vi "Object Node Tree.vi"(4 "Maximum Depth":i32=-1, 6 "Initial Path":string="$", 8 "error in (no error)":errorcluster, 10 "Offset":i32, 11 "JSON":string) -> (0 "error out":errorcluster, 1 "<JSON>":string[](array[string]) caption="<JSON>Items", 3 "$Paths":string[](array[string]))   [LabVIEW 2020]
doc: "Takes a JSON Value and \"flattens\" the Object structure, producing out arrays of the $Paths to each item and the corresponding items. This works recursively on all subObjects.\n\nNote: to support names containing periods (.) in them, those names will be retuurned as a JSON string (quoted). \n\nFor example: the JSON {\"A\":{\"B1\":1\"B2:\"x\"},\"A2\":true,\"A.1\":{\"C\":123}} produces the arrays:\n$Paths (Items):\n$.A.B1 (1)\n$.A.B2 (\"x\")\n$.A2 (true)\n$.\"A.1\".C (123)"
uses:
  <vilib>/JDP Science/JSONtext/JSONtext.lvlib
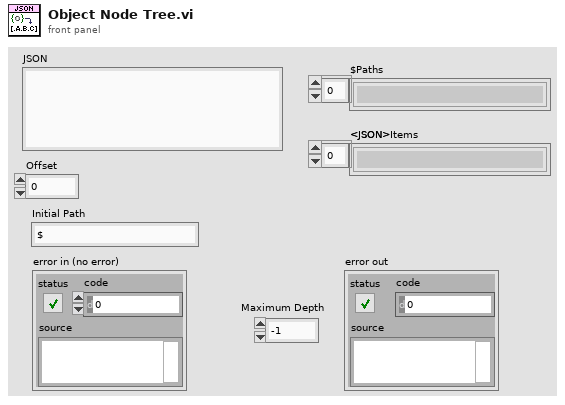
[diagram p1: front panel]
types:
  T1 = typedef "JSONtext.lvlib/JSON Value Type.ctl" = enum16{"Not a JSON Value", "JSON Object", "JSON Array", "String", "Number", "true", "false", "null"}
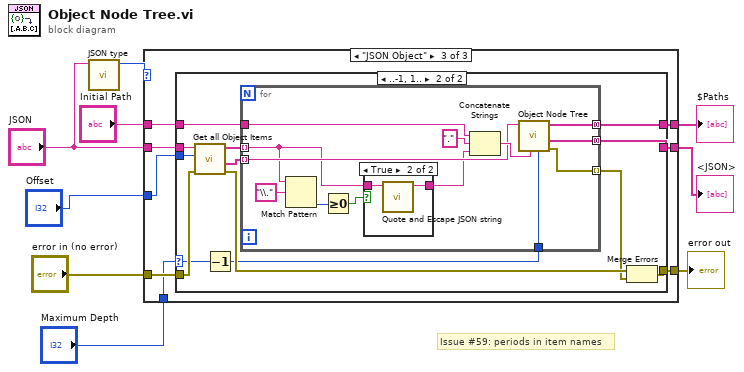
[diagram p0: block diagram]
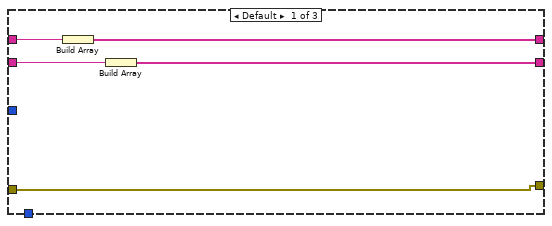
[diagram p2: hidden frame]
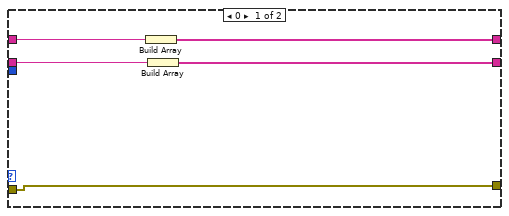
[diagram p4: hidden frame]
diagram:
  # "Issue #59: periods in item names"
  n1 = call <vilib>:"JSON type.vi"("JSON"="JSON") -> ("JSON Value Type"=w5:T1)  [unwired: 9 in, 1 out]
  n2 = case shown="\"JSON Object\"" w5 {
    tunnel: "JSON" -> [w14 _ w23]
    tunnel: [w11 _ w21] -> w6
    tunnel: [w13 _ w20] -> w7
    tunnel: "Initial Path" -> [w12 _ w22]
    tunnel: "Offset" -> [_ _ w19]
    tunnel: "error in (no error)" -> [w10 w15 w18]
    tunnel: [w10 w15 w17] -> w2
    tunnel: "Maximum Depth" -> [_ _ w16]
    frame Default {
      n3 = Build Array(w12) -> (w11:string[])
      n4 = Build Array(w14) -> (w13:string[])
    }
    frame "Not a JSON Value" {
    }
    frame "JSON Object" {
      n5 = case shown="..-1, 1.." w16 {
        selector: w16 -> [_ w30]
        tunnel: w23 -> [w26 w41]
        tunnel: w22 -> [w28 w40]
        tunnel: [w27 w39] -> w21
        tunnel: [w25 w36] -> w20
        tunnel: w19 -> [_ w35]
        tunnel: w18 -> [w24 w34]
        tunnel: [w24 w32] -> w17
        frame 0 {
          n6 = Build Array(w28) -> (w27:string[])
          n7 = Build Array(w26) -> (w25:string[])
        }
        frame ..-1, 1.. {
          n8 = call <vilib>:"Get all Object Items.vi"("error in (no error)"=w34, "Offset"=w35, "JSON"=w41) -> ("error out"=w33:errorcluster, "<JSON>"=w37:string[], "Item Names"=w38:string[])  [unwired: 5 in, 1 out]
          n9 = Decrement(x=w30) -> (x-1=w29:i32)
          n10 = for {
            tunnel: w40 -> [w54]
            tunnel: [w52] -> w39 mode=concatenating
            tunnel: w38 -> [w45] mode=indexing
            tunnel: w37 -> [w50] mode=indexing
            tunnel: [w49] -> w36 mode=concatenating
            tunnel: [w48] -> w31 mode=indexing
            tunnel: w29 -> [w42]
            n11 = Match Pattern(string=w45, regular expression="\\.") -> (offset past match=w46:i32)  [unwired: 1 in, 3 out]
            n12 = Greater Or Equal To 0?(x=w46) -> (x >= 0?=w43:bool)
            n13 = case shown="True" w43 {
              tunnel: w45 -> [w55 w57]
              tunnel: [w55 w56] -> w44
              frame False {
              }
              frame True {
                n14 = call <vilib>:"Quote and Escape JSON string.vi"("Plain Text"=w57) -> ("<JSON>"=w56:string)  [unwired: 10 in]
              }
            }
            n15 = Concatenate Strings(w54, "." ("string"), w44) -> (w51:string)
            n16 = call <vilib>:"Object Node Tree.vi"("Maximum Depth"=w42, "Initial Path"=w51, "JSON"=w50) -> ("error out"=w48:errorcluster, "<JSON>"=w49:string[], "$Paths"=w52:string[])  [unwired: 6 in]
          }
          n17 = Merge Errors(w33, w31) -> (w32:errorcluster)
        }
      }
    }
  }
  "<JSON>" <- w7
  "$Paths" <- w6
  "error out" <- w2
